vi "Reanimate.vi"(8 "Error In":errorcluster) -> (0 "Error Out":errorcluster)   [LabVIEW 2018, in "Tests.lvlib" / "Toolkit.lvlib" / "Integration.lvlib"]
uses:
  Integration.lvlib
  src/Toolkit/Toolkit.lvlib
  <vilib>/addons/_JKI Toolkits/Caraya/classes/Test/Test.lvclass
  <vilib>/addons/_JKI Toolkits/Caraya/classes/Assert/Assert.lvclass
  Tests.lvlib
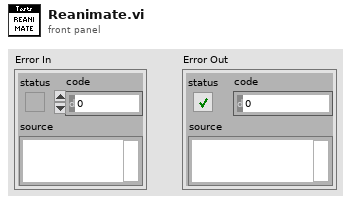
[diagram p1: front panel]
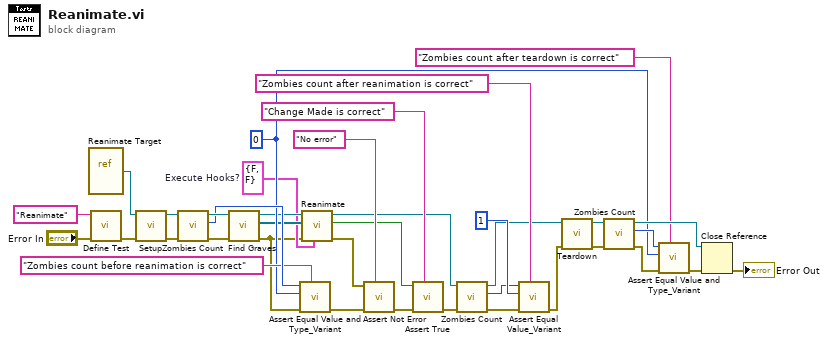
[diagram p0: block diagram]
diagram:
  w9 = cluster{"Pre":bool, "Post":bool} {"Pre"=FALSE, "Post"=FALSE}  # Execute Hooks?
  w13 = 0 ("size(s)")
  n1 = vi-ref "Reanimate Target.vi"() -> (w30:refnum<vi>)
  n2 = call <vilib>:"Define Test.vi"("error in (no error)"="Error In", "Label (VI Title)"="Reanimate") -> ("error out"=w28:errorcluster)  [unwired: 9 in]
  n3 = call "Setup.vi"("Error In"=w28, "VI In"=w30) -> ("Error Out"=w17:errorcluster, "VI Out"=w19:refnum<vi>)  [unwired: 8 in]
  n4 = call "Zombies Count.vi"("Error In"=w17, "Test Target In"=w19) -> ("Error Out"=w20:errorcluster, "Zombies Count"=w16:i32, "Test Target Out"=w18:refnum<vi>)  [unwired: 7 in]
  n5 = call "Find Graves.vi"("Error In"=w20, "VI In"=w18) -> ("Error Out"=w8:errorcluster, "Graves"=w11:refnum<vi>[], "VI Out"=w12:refnum<vi>)  [unwired: 7 in]
  n6 = call <vilib>:"Assert Equal Value and Type_Variant.vi"("Label"="Zombies count before reanimation is correct", "error in (no error)"=w8, "Y"=w13, "X"=w16) -> ("error out"=w14:errorcluster)  [unwired: 7 in]
  n7 = call "Reanimate.vi"("Execute Hooks?"=w9, "Error In"=w8, "Graves"=w11, "VI In"=w12) -> ("Error Out"=w7:errorcluster, "Change Made?"=w10:bool, "VI Out"=w3:refnum<vi>)  [unwired: 5 in]
  n8 = call <vilib>:"Assert Not Error.vi"("Label"="No error", "error in (no error)"=w14, "Not Error?"=w7) -> ("error out"=w35:errorcluster)  [unwired: 8 in]
  n9 = call <vilib>:"Assert True.vi"("Label"="Change Made is correct", "error in (no error)"=w35, "True?"=w10) -> ("error out"=w6:errorcluster)  [unwired: 8 in]
  n10 = call "Zombies Count.vi"("Error In"=w6, "Test Target In"=w3) -> ("Error Out"=w5:errorcluster, "Zombies Count"=w1:i32, "Test Target Out"=w2:refnum<vi>)  [unwired: 7 in]
  n11 = call <vilib>:"Assert Equal Value_Variant.vi"("Label"="Zombies count after reanimation is correct", "error in (no error)"=w5, "Y"=1 ("size(s)"), "X"=w1) -> ("error out"=w4:errorcluster)  [unwired: 7 in]
  n12 = call "Teardown.vi"("Error In"=w4, "VI In"=w2) -> ("Error Out"=w26:errorcluster, "VI Out"=w27:refnum<vi>)  [unwired: 8 in]
  n13 = call "Zombies Count.vi"("Error In"=w26, "Test Target In"=w27) -> ("Error Out"=w25:errorcluster, "Zombies Count"=w21:i32, "Test Target Out"=w23:refnum<vi>)  [unwired: 7 in]
  n14 = call <vilib>:"Assert Equal Value and Type_Variant.vi"("Label"="Zombies count after teardown is correct", "error in (no error)"=w25, "Y"=w13, "X"=w21) -> ("error out"=w24:errorcluster)  [unwired: 7 in]
  n15 = Close Reference(reference=w23, error in (no error)=w24) -> (error out=→"Error Out":errorcluster)
